vi "test-trajectory-generator-JAS-CONSTRAINT-PLAY.vi"() -> (3 "Okay":bool)   [LabVIEW 2019]
uses:
  <vilib>/Rock Robotics/SystemInterfaces/NetworkCommunication/NetComm_UsageReport_report.vi
  <vilib>/Rock Robotics/WPI/ThirdParty/JAS_Junk/TrajLib/DiffDriveKinematicsConstraint_New.vi
  <vilib>/Rock Robotics/WPI/ThirdParty/JAS_Junk/TrajLib/Util_LibraryGlobals.vi
  <vilib>/Rock Robotics/WPI/ThirdParty/JAS_Junk/TrajLib/Trajectory_Library.lvlib
panel:
  in  "Use Accel":bool
  out "Wheel Acceleration":cluster{dbl[], dbl[]}[](graph)
  out "Wheel velocity":cluster{dbl[], dbl[]}[](graph)
  out "Chassis Info":cluster{dbl[], dbl[]}[](graph)
  out "XY Graph":cluster{dbl[], dbl[]}(graph)
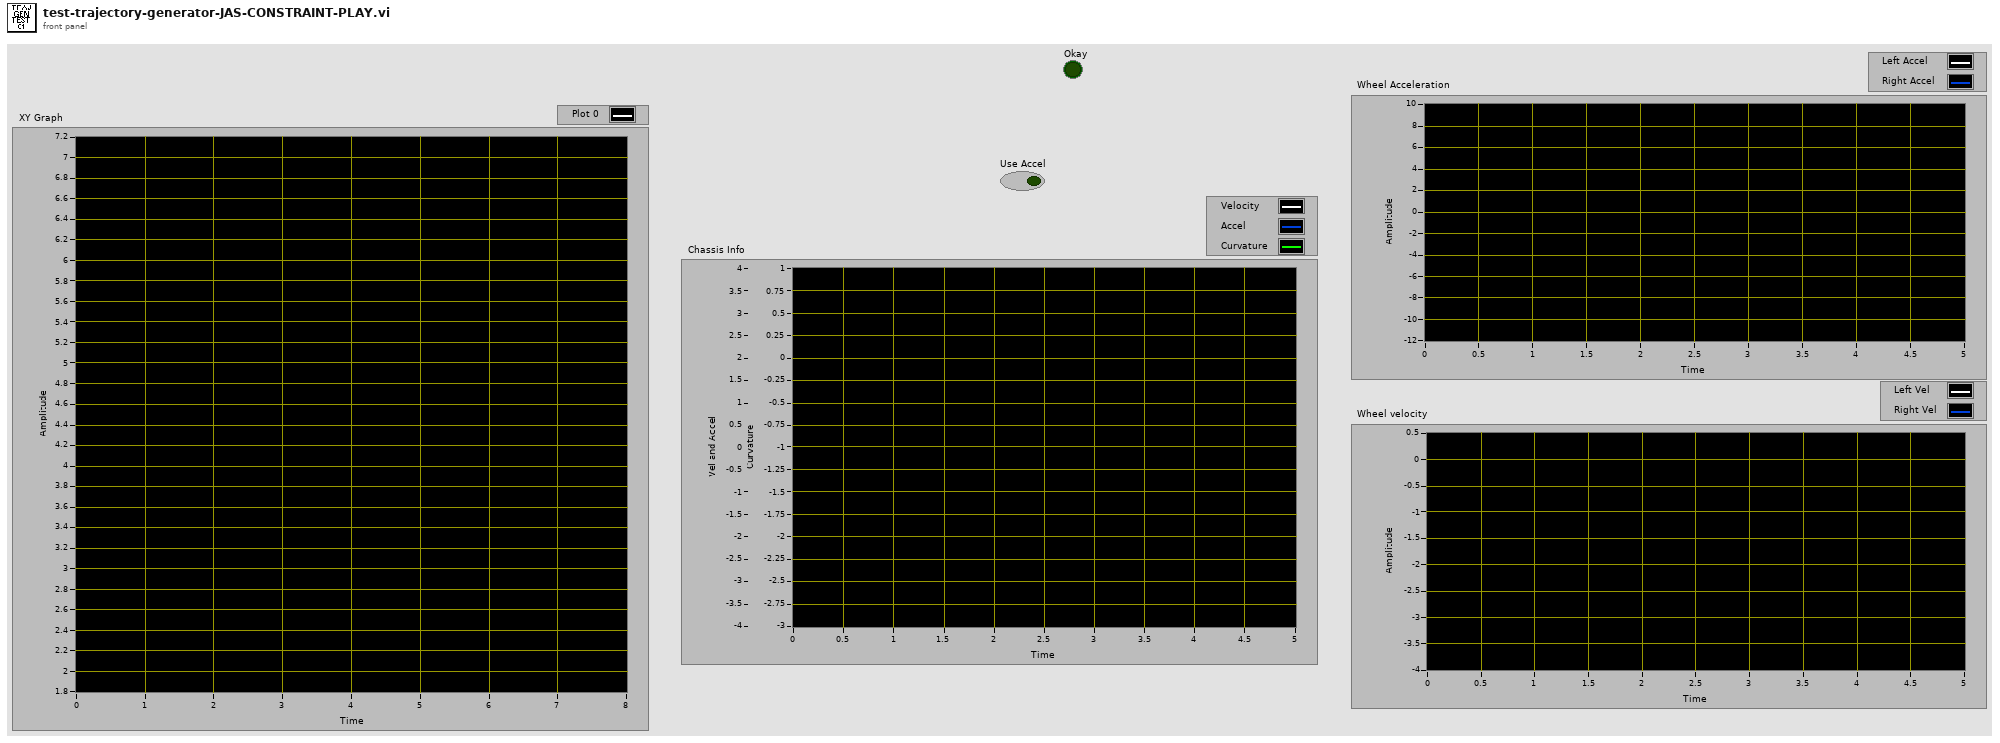
[diagram p1: front panel]
types:
  T1 = typedef "Trajectory_Library.lvlib/TRAJ_CONFIG.ctl" = cluster{"MaxVelocity":dbl, "Max Acceleration":dbl, "StartVelocity":dbl, "End Velocity":dbl, "Reversed":bool, "DiffDrKineConstntDefined":bool, "CentAcellConstntDefined":bool, "DiffDrVoltConstntDefined":bool, "DIFF_DRIVE_KINE_CONSTRAINT":T2, "CENTRIPETAL_ACCEL_CONSTRAINT":T4, "SwerveDrKineConstntDefined":bool, "SWERVE_DRIVE_KINE_CONSTRAINT":T5, "DIFF_DRIVE_VOLTAGE_CONSTRAINT":T9, "MECANUM_DRIVE_KINE_CONSTRAINT":T11, "MecanumDrKineConstntDefined":bool}
  T2 = typedef "Trajectory_Library.lvlib/TRAJ_CONSTRAINT_DIIF_DRIVE_KINEMATICS.ctl" = cluster{"Max Speed (M/S)":dbl, "DIFF_DRIVE_KINEMATICS":T3, "Max Accel (M/S2)":dbl}
  T3 = typedef "Trajectory_Library.lvlib/DIFF_DRIVE_KINEMATICS.ctl" = cluster{"TrackWidth_Meters":dbl}
  T4 = typedef "Trajectory_Library.lvlib/TRAJ_CONSTRAINT_CENTRIPETAL_ACCEL.ctl" = cluster{"Max Cent Accel":dbl}
  T5 = typedef "Trajectory_Library.lvlib/TRAJ_CONSTRAINT_SWERVE_DRIVE_KINEMATICS.ctl" = cluster{"Max Speed (M/S)":dbl, "SwerveKinematics":T6}
  T6 = typedef "Trajectory_Library.lvlib/SWERVE_DRIVE_KINEMATICS.ctl" = cluster{"NumModules":i32, "InverseKinematics":T7, "ForwardKinematics":T7, "Modules":T8[], "PrevCoR":T8}
  T7 = typedef "NI_Matrix.lvlib/RealMatrix.ctl" = dbl[][]
  T8 = typedef "Trajectory_Library.lvlib/TRANSLATION2D.ctl" = cluster{"X":dbl, "Y":dbl}
  T9 = typedef "Trajectory_Library.lvlib/TRAJ_CONSTRAINT_DIIF_DRIVE_VOLTAGE.ctl" = cluster{"Max Voltage":dbl, "DIFF_DRIVE_KINEMATICS":T3, "SIMPLE_MOTOR_FF":T10}
  T10 = typedef "Trajectory_Library.lvlib/SIMPLE_MOTOR_FF.ctl" = cluster{"Ks":dbl, "Kv":dbl, "Ka":dbl}
  T11 = typedef "Trajectory_Library.lvlib/TRAJ_CONSTRAINT_MECA_DRIVE_KINEMATICS.ctl" = cluster{"Max Speed (M/S)":dbl, "MECA_DRIVE_KINEMATICS":T12}
  T12 = typedef "Trajectory_Library.lvlib/MECA_DRIVE_KINEMATICS.ctl" = cluster{"FrontLeft":T8, "FrontRight":T8, "RearLeft":T8, "RearRight":T8, "InverseKinematics":T7, "ForwardKinematics":T7, "PrevCoR":T8}
  T13 = typedef "Trajectory_Library.lvlib/TRAJECTORY.ctl" = cluster{"TotalTImeSecs":dbl, "States":T14[]}
  T14 = typedef "Trajectory_Library.lvlib/TRAJ_STATE.ctl" = cluster{"TimeSeconds":dbl, "Velocity":dbl, "Acceleration":dbl, "POSE":T15, "Curvature":dbl}
  T15 = typedef "Trajectory_Library.lvlib/POSE2D.ctl" = cluster{"TRANSLATION":T8, "ROTATION":T16}
  T16 = typedef "Trajectory_Library.lvlib/ROTATION2D.ctl" = cluster{"VALUE":dbl, "COS":dbl, "SIN":dbl}
  T17 = typedef "Trajectory_Library.lvlib/CHASSIS_SPEEDS.ctl" = cluster{"vX":dbl, "vY":dbl, "vOmega":dbl}
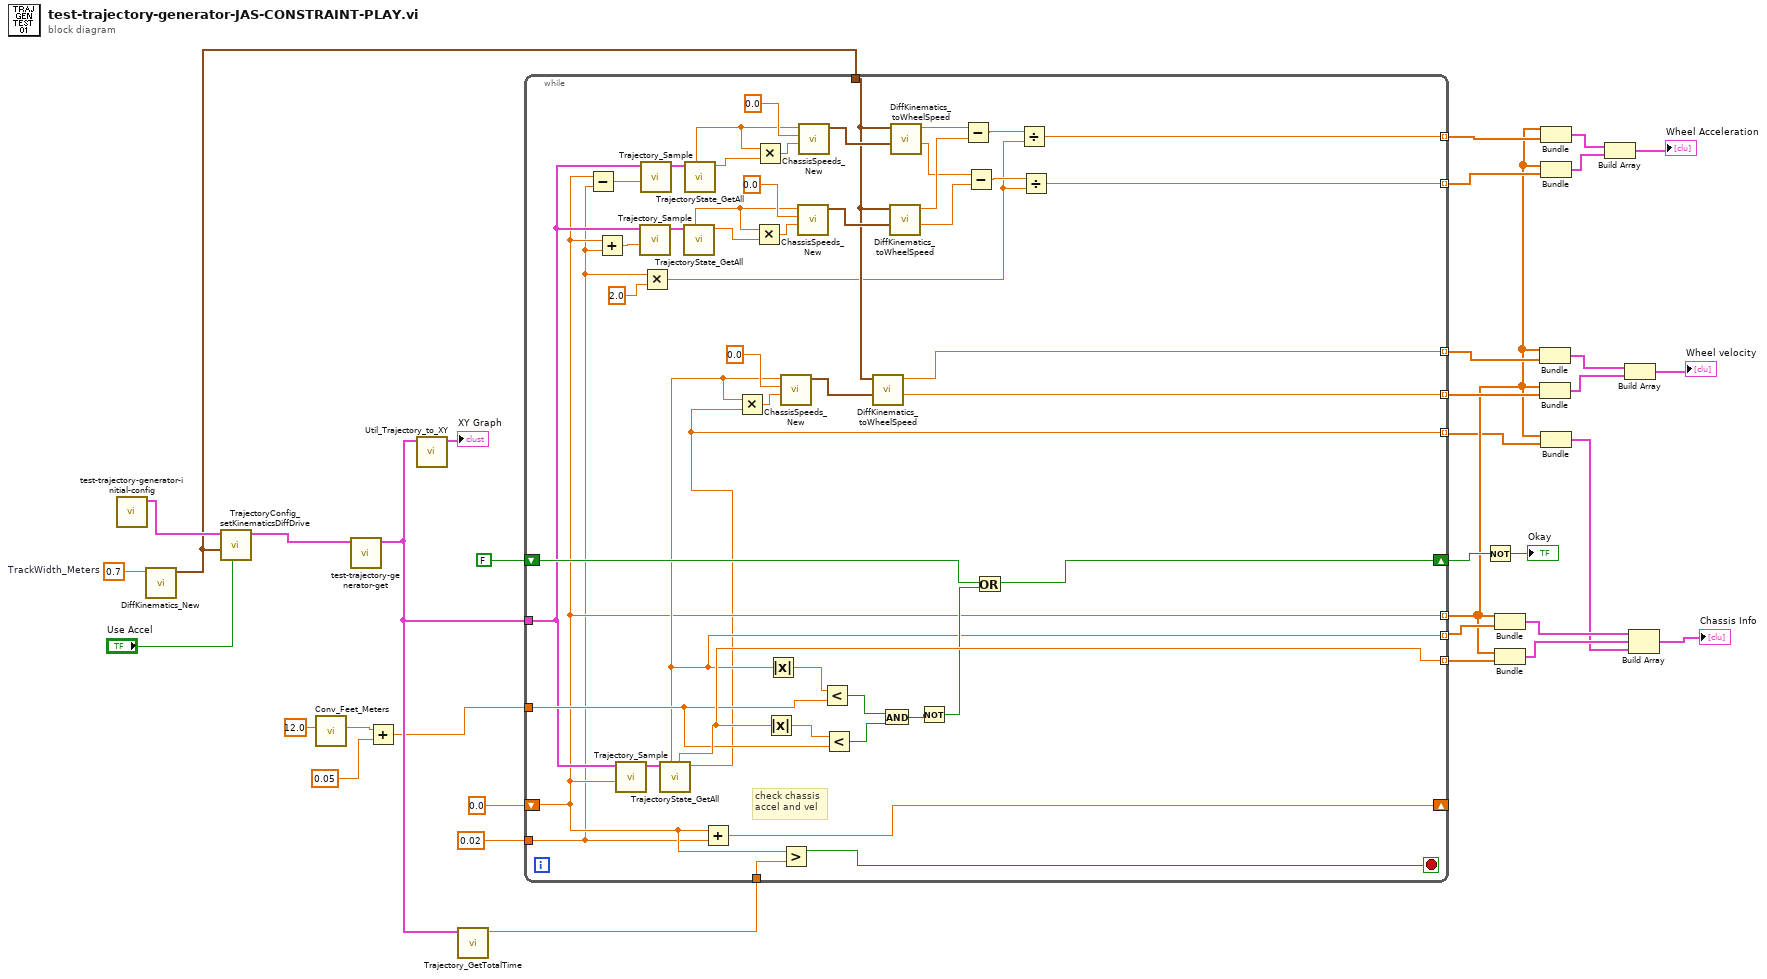
[diagram p0: block diagram]
diagram:
  w18 = 0.7  # TrackWidth_Meters
  n1 = call "test-trajectory-generator-initial-config.vi"() -> ("traj_config"=w17:T1)  [unwired: 11 in]
  n2 = call <vilib>:"DiffKinematics_New.vi"("TrackWidth_Meters"=w18) -> ("DIFF_DRIVE_KINEMATICS"=w15:T3)  [unwired: 10 in]
  n3 = call <vilib>:"TrajectoryConfig_setKinematicsDiffDrive.vi"("Use Accel"="Use Accel", "DIFF_DRIVE_KINEMATICS"=w15, "inTRAJECTORY_CONFIG"=w17) -> ("outTRAJECTORY_CONFIG"=w16:T1)  [unwired: 8 in]
  n4 = call <vilib>:"Conv_Feet_Meters.vi"("Feet"=12.0) -> ("Meters"=w21:dbl)  [unwired: 10 in]
  n5 = call "test-trajectory-generator-get.vi"("traj_config"=w16) -> ("TRAJECTORY"=w24:T13)  [unwired: 8 in, 2 out]
  n6 = Add(x=w21, y=0.05) -> (x+y=w19:dbl)
  n7 = call <vilib>:"Util_Trajectory_to_XY.vi"("TRAJECTORY"=w24) -> ("outArrayXY"=→"XY Graph":cluster{dbl[], dbl[]})  [unwired: 10 in]
  n8 = call <vilib>:"Trajectory_GetTotalTime.vi"("TRAJECTORY"=w24) -> ("TotalTime_Sec"=w23:dbl)  [unwired: 10 in]
  n9 = while {
    tunnel: 0.02 -> [w43]
    shift-right: [w74] -> _
    shift-left: 0.0 -> [w61]
    tunnel: w24 -> [w62]
    tunnel: [w68] -> w32 mode=indexing
    tunnel: [w80] -> w31 mode=indexing
    tunnel: [w61] -> w4 mode=indexing
    shift-right: [w75] -> w26
    shift-left: FALSE -> [w75]
    tunnel: w23 -> [w73]
    tunnel: w19 -> [w71]
    tunnel: w15 -> [w52]
    tunnel: [w66] -> w12 mode=indexing
    tunnel: [w65] -> w11 mode=indexing
    tunnel: [w38] -> w6 mode=indexing
    tunnel: [w37] -> w5 mode=indexing
    tunnel: [w36] -> w3 mode=indexing
    stop <- w72 stop-if-true
    # "check chassis\naccel and vel"
    n10 = Subtract(x=w61, y=w43) -> (x-y=w60:dbl)
    n11 = Add(x=w61, y=w43) -> (x+y=w59:dbl)
    n12 = call <vilib>:"Trajectory_Sample.vi"("Time"=w61, "InputTRAJECTORY"=w62) -> ("OutputTRAJ_STATE"=w83:T14)  [unwired: 9 in]
    n13 = call <vilib>:"Trajectory_Sample.vi"("Time"=w59, "InputTRAJECTORY"=w62) -> ("OutputTRAJ_STATE"=w63:T14)  [unwired: 9 in]
    n14 = call <vilib>:"Trajectory_Sample.vi"("Time"=w60, "InputTRAJECTORY"=w62) -> ("OutputTRAJ_STATE"=w64:T14)  [unwired: 9 in]
    n15 = Multiply(x=w43, y=2.0) -> (x*y=w39:dbl)
    n16 = call <vilib>:"TrajectoryState_GetAll.vi"("TRAJ_STATE"=w83) -> ("Curvature"=w36:dbl, "Acceleration"=w80:dbl, "Velocity"=w68:dbl)  [unwired: 4 in, 4 out]
    n17 = call <vilib>:"TrajectoryState_GetAll.vi"("TRAJ_STATE"=w63) -> ("Curvature"=w49:dbl, "Velocity"=w50:dbl)  [unwired: 4 in, 5 out]
    n18 = call <vilib>:"TrajectoryState_GetAll.vi"("TRAJ_STATE"=w64) -> ("Curvature"=w48:dbl, "Velocity"=w51:dbl)  [unwired: 4 in, 5 out]
    n19 = Add(x=w61, y=w43) -> (x+y=w74:dbl)
    n20 = Multiply(x=w68, y=w36) -> (x*y=w69:dbl)
    n21 = Multiply(x=w50, y=w49) -> (x*y=w54:dbl)
    n22 = Multiply(x=w51, y=w48) -> (x*y=w57:dbl)
    n23 = Absolute Value(x=w80) -> (abs(x)=w81:dbl)
    n24 = Absolute Value(x=w68) -> (abs(x)=w82:dbl)
    n25 = call <vilib>:"ChassisSpeeds_New.vi"("vAngular"=w69, "vY"=0.0, "vX"=w68) -> ("CHASSIS"=w67:T17)  [unwired: 8 in]
    n26 = Greater?(x=w61, y=w73) -> (0:w72:bool)
    n27 = call <vilib>:"ChassisSpeeds_New.vi"("vAngular"=w54, "vY"=0.0, "vX"=w50) -> ("CHASSIS"=w53:T17)  [unwired: 8 in]
    n28 = call <vilib>:"ChassisSpeeds_New.vi"("vAngular"=w57, "vY"=0.0, "vX"=w51) -> ("CHASSIS"=w56:T17)  [unwired: 8 in]
    n29 = Less?(x=w82, y=w71) -> (x < y?=w79:bool)
    n30 = Less?(x=w81, y=w71) -> (x < y?=w78:bool)
    n31 = call <vilib>:"DiffKinematics_toWheelSpeed.vi"("CHASSIS Speed"=w67, "DIFF_DRIVE_KINEMATICS"=w52) -> ("RightVelocity"=w65:dbl, "LeftVelocity"=w66:dbl)  [unwired: 8 in]
    n32 = And(x=w79, y=w78) -> (x .and. y?=w77:bool)
    n33 = call <vilib>:"DiffKinematics_toWheelSpeed.vi"("CHASSIS Speed"=w53, "DIFF_DRIVE_KINEMATICS"=w52) -> ("RightVelocity"=w44:dbl, "LeftVelocity"=w46:dbl)  [unwired: 8 in]
    n34 = call <vilib>:"DiffKinematics_toWheelSpeed.vi"("CHASSIS Speed"=w56, "DIFF_DRIVE_KINEMATICS"=w52) -> ("RightVelocity"=w45:dbl, "LeftVelocity"=w47:dbl)  [unwired: 8 in]
    n35 = Not(x=w77) -> (.not. x?=w76:bool)
    n36 = Subtract(x=w47, y=w46) -> (x-y=w40:dbl)
    n37 = Subtract(x=w45, y=w44) -> (x-y=w41:dbl)
    n38 = Or(x=w75, y=w76) -> ()  [unwired: 1 out]
    n39 = Divide(x=w40, y=w39) -> (x/y=w38:dbl)
    n40 = Divide(x=w41, y=w39) -> (x/y=w37:dbl)
  }
  n41 = Not(x=w26) -> (.not. x?=→"Okay":bool)
  n42 = Bundle(w4, w32) -> (w30:cluster{dbl[], dbl[]})  [unwired: 1 in]
  n43 = Bundle(w4, w31) -> (w29:cluster{dbl[], dbl[]})  [unwired: 1 in]
  n44 = Bundle(w4, w12) -> (w14:cluster{dbl[], dbl[]})  [unwired: 1 in]
  n45 = Bundle(w4, w11) -> (w13:cluster{dbl[], dbl[]})  [unwired: 1 in]
  n46 = Bundle(w4, w6) -> (w9:cluster{dbl[], dbl[]})  [unwired: 1 in]
  n47 = Bundle(w4, w5) -> (w8:cluster{dbl[], dbl[]})  [unwired: 1 in]
  n48 = Bundle(w4, w3) -> (w2:cluster{dbl[], dbl[]})  [unwired: 1 in]
  n49 = Build Array(w9, w8) -> (→"Wheel Acceleration":cluster{dbl[], dbl[]}[])
  n50 = Build Array(w14, w13) -> (→"Wheel velocity":cluster{dbl[], dbl[]}[])
  n51 = Build Array(w30, w29, w2) -> (→"Chassis Info":cluster{dbl[], dbl[]}[])
